vi "I2C_Init.vi"(10 "DevType":i32) -> (1 "LedSensorInit":bool)   [LabVIEW 2017]
uses:
  jtool.dll
panel:
  out "s? t:f":string
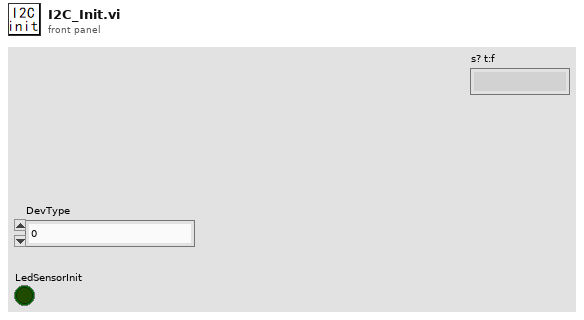
[diagram p1: front panel]
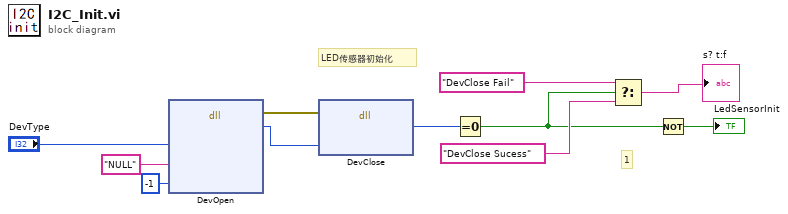
[diagram p0: block diagram]
diagram:
  # "1"
  # "LED传感器初始化"
  n1 = dll-call lib="D:/X682 Camera Calibration Tester Program/HardWare/Led_I2C2561/jtool.dll" fn="DevOpen"("DevType"="DevType", "Sn"="NULL", "Id"=-1) -> (error out=w6:errorcluster, "返回类型"=w5:i32)  [unwired: 6 in, 1 out]
  n2 = dll-call lib="D:/X682 Camera Calibration Tester Program/HardWare/Led_I2C2561/jtool.dll" fn="DevClose"(error in=w6, "DevHandle"=w5) -> ("返回类型"=w9:u8)  [unwired: 3 in, 2 out]
  n3 = Equal To 0?(x=w9) -> (x = 0?=w4:bool)
  n4 = Select(t="DevClose Fail", s=w4, f="DevClose Sucess") -> (s? t:f=→"s? t:f":string)
  n5 = Not(x=w4) -> (.not. x?=→"LedSensorInit":bool)
